vi "mWtoWatts.vi"(1 "mW":dbl) -> (0 "W":dbl)   [LabVIEW 2015]
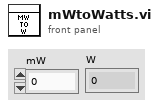
[diagram p1: front panel]
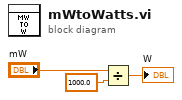
[diagram p0: block diagram]
diagram:
  n1 = Divide(x="mW", y=1000.0) -> (x/y=→"W":dbl)
